vi "Create Expression to Update Test Limits.vi"(8 "Error In":errorcluster, 10 "All_Limits":string[][](array[string])=[["TestName", "Key", "TestNumber", "Low Limit", "High Limit", "TestStand Test Name", "", "", ""], ["IVIOKGD", "Start", "1", "0", "3", "IVSU_LowPower_Initial", "", "", ""], ["", "End", "2", "50", "100", "IVSU_State0x00_Initial", "", "", ""], ["", "", "", "", "", "", "", "", "`"], ["Initial_States", "Start", "1", "50", "100", "IVSU_State0x0F_Initial", "", "", ""], ["", "End", "2", "50", "100", "IVSU_State0xF0_Initial", "", "", ""], ["", "", "", "", "", "", "", "", ""], ["Rfree_Initial", "Start", "1", "395k", "3M", "RF1", "", "", ""], ["", "", "2", "395k", "3M", "RF2", "", "", ""], ["", "", "3", "445k", "3M", "RF3", "", "", ""], ["", "End", "4", "445k", "3M", "RF4", "", "", ""], ["", "", "", "", "", "", "", "", ""], ["Ron_Initial", "Start", "1", "0.35", "2", "RF1", "", "", ""], ["", "", "2", "0.35", "2", "RF2", "", "", ""], ["", "", "3", "0.35", "2", "RF3", "", "", ""], ["", "End", "4", "0.35", "2", "RF4", "", "", ""], ["", "", "", "", "", "", "", "", ""], ["Ron_Conditioned", "Start", "1", "0.35", "1", "RF1", "", "", ""], ["", "", "2", "0.35", "1", "RF2", "", "", ""], ["", "", "3", "0.35", "1", "RF3", "", "", ""], ["", "End", "4", "0.35", "1", "RF4", "", "", ""], ["", "", "", "", "", "", "", "", ""], ["Butterfly", "Start", "55", "33", "39", "R_VPI", "", "", ""], ["", "End", "56", "30", "39", "R_VRL", "", "", ""], ["", "", "", "", "", "", "", "", ""], ["Rshunt", "Start", "1", "10", "20", "Rshunt_RF1", "", "", ""], ["", "", "2", "10", "20", "Rshunt_RF2", "", "", ""], ["", "", "3", "10", "20", "Rshunt_RF3", "", "", ""], ["", "End", "4", "10", "20", "Rshunt_RF4", "", "", ""], ["", "", "", "", "", "", "", "", ""], ["Guardian", "Start", "1", "1", "5", "GuardianPilot_On", "", "", ""], ["", "End", "2", "175k", "225k", "GuardianPilot_Off", "", "", ""], ["", "", "", "", "", "", "", "", ""], ["Final_States", "Start", "1", "50", "100", "IVSU_State0x0F_Final", "", "", ""], ["", "End", "2", "50", "100", "IVSU_State0xF0_Final", "", "", ""], ["", "", "", "", "", "", "", "", ""], ["Rfree_Final", "Start", "1", "395k", "445k", "RF1", "", "", ""], ["", "", "2", "395k", "445k", "RF2", "", "", ""], ["", "", "3", "445k", "495k", "RF3", "", "", ""], ["", "End", "4", "445k", "495k", "RF4", "", "", ""], ["", "", "", "", "", "", "", "", ""], ["", "", "", "", "", "", "", "", ""], ["Reverse_IVIOKGD", "Start", "1", "50", "100", "IVSU_State0x00_Final", "", "", ""], ["", "End", "2", "0", "3", "IVSU_LowPower_Final", "", "", ""]], 11 "Test Name":string="IVIOKGD") -> (0 "Error Out":errorcluster, 3 "Limits_Expression":string)   [LabVIEW 2013]
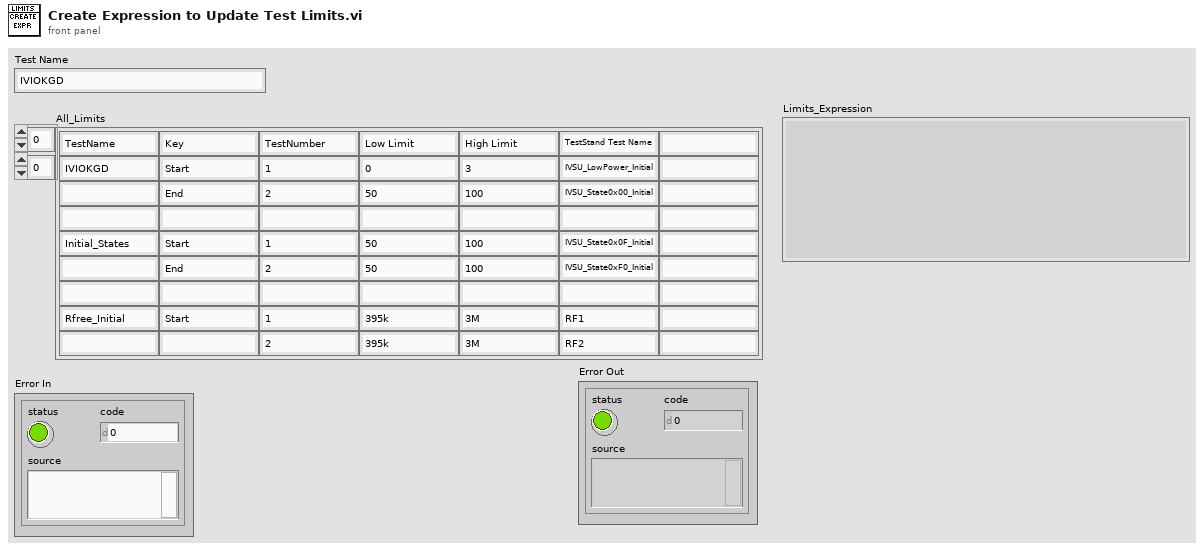
[diagram p1: front panel]
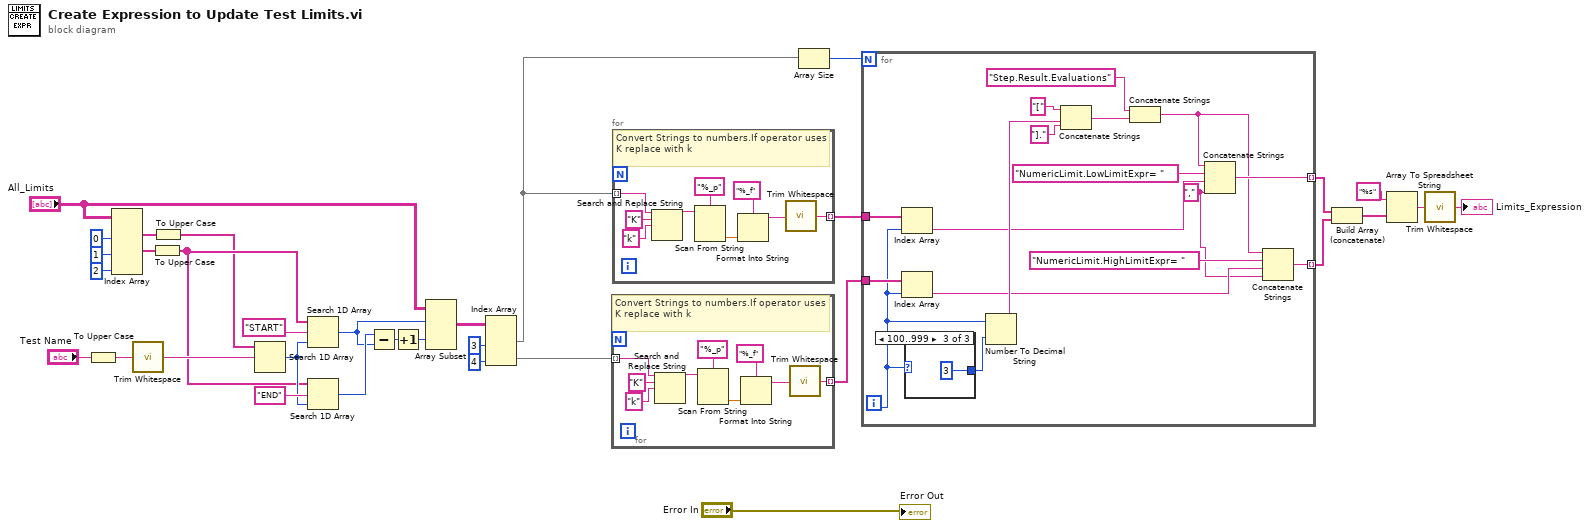
[diagram p0: block diagram]
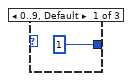
[diagram p2: hidden frame]
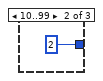
[diagram p3: hidden frame]
diagram:
  n1 = To Upper Case(1:"Test Name") -> (0:w29:string)
  n2 = Index Array(array="All_Limits", index (col) #1=0 ("disabled index (col)"), index (col) #2=1 ("index (col)"), index (col) #3=2 ("index (col)")) -> (element #1=w16:string[], element #2=w18:string[])  [unwired: 3 in, 1 out]
  n3 = call <vilib>:"Trim Whitespace.vi"("string"=w29) -> ("trimmed string"=w27:string)  [unwired: 1 in]
  n4 = To Upper Case(1:w18) -> (0:w17:string[])
  n5 = To Upper Case(1:w16) -> (0:w15:string[])
  n6 = Search 1D Array(1D array=w15, element=w27) -> (index of element=w21:i32)  [unwired: 1 in]
  n7 = Search 1D Array(1D array=w17, element="START", start index (0)=w21) -> (index of element=w19:i32)
  n8 = Search 1D Array(1D array=w17, element="END", start index (0)=w21) -> (index of element=w24:i32)
  n9 = Subtract(x=w24, y=w19) -> (x-y=w23:i32)
  n10 = Increment(x=w23) -> (x+1=w22:i32)
  n11 = Array Subset(array="All_Limits", index (row)=w19, length (row)=w22) -> (w20:string[][])  [unwired: 2 in]
  n12 = Index Array(array=w20, index (col) #1=3 ("index (col)"), index (col) #2=4 ("index (col)")) -> (element #1=w12:string[], element #2=w10:string[])  [unwired: 2 in]
  n13 = for {
    tunnel: w10 -> [w41] mode=indexing
    tunnel: [w34] -> w9 mode=indexing
    # "Convert Strings to numbers.If operator uses K replace with k"
    n14 = Search and Replace String(input string=w41, search string="K", replace string="k" ("search string")) -> (result string=w39:string)  [unwired: 5 in, 3 out]
    n15 = Scan From String(format string="%_p", input string=w39) -> (output 1=w36:dbl)  [unwired: 3 in, 3 out]
    n16 = Format Into String(format string="%_f", w36) -> (resulting string=w35:string)  [unwired: 2 in, 1 out]
    n17 = call <vilib>:"Trim Whitespace.vi"("string"=w35) -> ("trimmed string"=w34:string)  [unwired: 1 in]
  }
  n18 = for {
    tunnel: w12 -> [w50] mode=indexing
    tunnel: [w43] -> w11 mode=indexing
    # "Convert Strings to numbers.If operator uses K replace with k"
    n19 = Search and Replace String(input string=w50, search string="K", replace string="k" ("search string")) -> (result string=w48:string)  [unwired: 5 in, 3 out]
    n20 = Scan From String(format string="%_p", input string=w48) -> (output 1=w45:dbl)  [unwired: 3 in, 3 out]
    n21 = Format Into String(format string="%_f", w45) -> (resulting string=w44:string)  [unwired: 2 in, 1 out]
    n22 = call <vilib>:"Trim Whitespace.vi"("string"=w44) -> ("trimmed string"=w43:string)  [unwired: 1 in]
  }
  n23 = Array Size(array=w12) -> (size(s)=w4:i32)
  n24 = for {
    N: w4 -> [_]
    tunnel: w9 -> [w62]
    tunnel: w11 -> [w59]
    tunnel: [w57] -> w6 mode=indexing
    tunnel: [w52] -> w5 mode=indexing
    i -> [w61]
    w53 = "," ("string")
    n25 = Index Array(array=w59, index=w61) -> (element=w58:string)
    n26 = Index Array(array=w62, index=w61) -> (element=w54:string)
    n27 = case shown="100..999" w61 {
      tunnel: [i16 1 ("width (-)") i16 2 ("width (-)") i16 3 ("width (-)")] -> w68
      frame 0..9, Default {
      }
      frame 10..99 {
      }
      frame 100..999 {
      }
    }
    n28 = Number To Decimal String(number=w61, width (-)=w68) -> (decimal integer string=w63:string)
    n29 = Concatenate Strings("[", w63, "].") -> (w64:string)
    n30 = Concatenate Strings("Step.Result.Evaluations", w64) -> (w56:string)
    n31 = Concatenate Strings(w56, "NumericLimit.LowLimitExpr= ", w58, w53) -> (w57:string)
    n32 = Concatenate Strings(w56, "NumericLimit.HighLimitExpr= ", w54, w53) -> (w52:string)
  }
  n33 = Build Array (concatenate)(w6, w5) -> (w7:string[])
  n34 = Array To Spreadsheet String(array=w7, 3:"%s" ("format string")) -> (spreadsheet string=w3:string)  [unwired: 1 in]
  n35 = call <vilib>:"Trim Whitespace.vi"("string"=w3) -> ("trimmed string"=→"Limits_Expression":string)  [unwired: 1 in]
  "Error Out" <- "Error In"
